vi "GetAverageDataInSpecifiedTime.vi"(8 "error in (no error)":errorcluster caption="错误输入（无错误）", 10 "DataIn":waveform(dbl)[](array[waveform]), 11 "SelectPointObj 输入":refnum<class "SelectPointObj.lvclass"> caption="DNL_LabVIEW Object in") -> (0 "error out":errorcluster caption="错误输出", 3 "SelectPointObj 输出":refnum<class "SelectPointObj.lvclass"> caption="DNL_LabVIEW Object out")   [LabVIEW 2016, in "SelectPointObj.lvclass"]
uses:
  SelectPointObj.lvclass
  SelectPointObj.lvclass/SelectPointObj.ctl
  <vilib>/Analysis/baseanly.llb/Mean (DBL).vi
  <vilib>/Analysis/NI_AALBase.lvlib
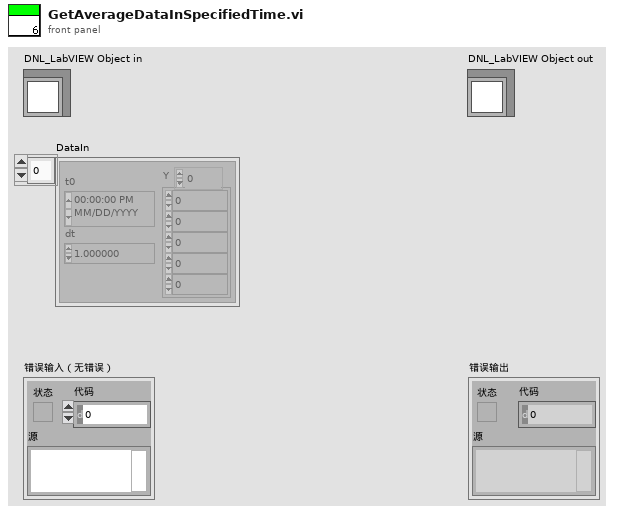
[diagram p1: front panel]
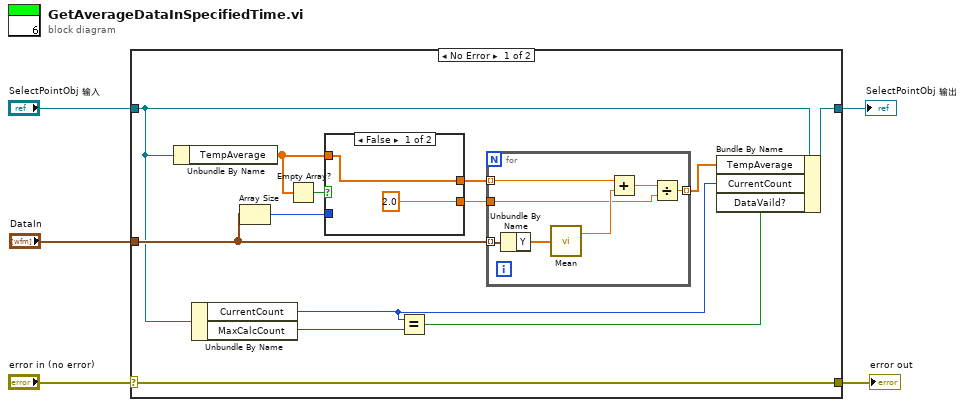
[diagram p0: block diagram]
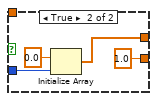
[diagram p2: hidden frame]
diagram:
  n1 = case shown="No Error" "error in (no error)" {
    selector: "error in (no error)" -> [w18 w33]
    tunnel: [w18 w33] -> w4
    tunnel: [w17 w32] -> w2
    tunnel: "SelectPointObj 输入" -> [w10 w32]
    tunnel: "DataIn" -> [w16 _]
    frame No Error {
      n2 = Unbundle By Name(w10) -> ("TempAverage"=w11:dbl[])
      n3 = Unbundle By Name(w10) -> ("CurrentCount"=w7:i32, "MaxCalcCount"=w9:i32)
      n4 = Array Size(array=w16) -> (size(s)=w14:i32)
      n5 = Empty Array?(array=w11) -> (empty?=w12:bool)
      n6 = case shown="False" w12 {
        tunnel: w14 -> [_ w23]
        tunnel: [w20 w22] -> w13
        tunnel: w11 -> [w20 _]
        tunnel: [2.0 1.0] -> w6
        frame False {
        }
        frame True {
          n7 = Initialize Array(0.0, w23) -> (w22:dbl[])
        }
      }
      n8 = Equal?(x=w7, y=w9) -> (x = y?=w8:bool)
      n9 = for {
        tunnel: w16 -> [w31] mode=indexing
        tunnel: [w27] -> w15 mode=indexing
        tunnel: w13 -> [w26] mode=indexing
        tunnel: w6 -> [w25]
        n10 = Unbundle By Name(w31) -> ("Y"=w30:dbl[])
        n11 = call-poly <vilib>:"Mean.vi"("X"=w30) -> ("mean"=w28:dbl)  [unwired: 1 out]
        n12 = Add(x=w26, y=w28) -> (x+y=w29:dbl)
        n13 = Divide(x=w29, y=w25) -> (x/y=w27:dbl)
      }
      n14 = Bundle By Name(cluster=w10, "TempAverage"=w15, "CurrentCount"=w7, "DataVaild?"=w8) -> (w17:refnum<class "SelectPointObj.lvclass">)
    }
    frame Error {
    }
  }
  "error out" <- w4
  "SelectPointObj 输出" <- w2
